vi "2D Array to Excel 2012.vi"   [LabVIEW 2012]
uses:
  <vilib>/Utility/NIReport.llb/NI_report.lvclass
  <vilib>/Utility/NIReport.llb/Excel/NI_Excel.lvclass
  <vilib>/Utility/NIReport.llb/Append Numeric Table to Report (wrap).vi
types:
  T1 = enum16{"Standard Report", "HTML", "Word", "Excel"}
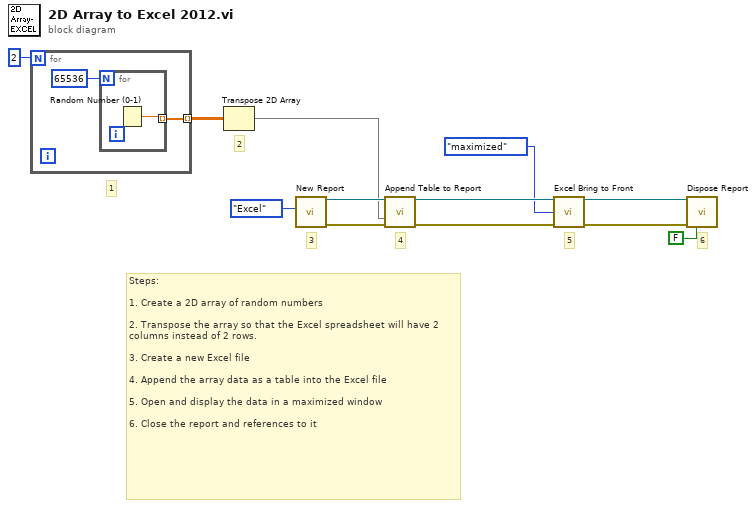
[diagram p0: block diagram]
diagram:
  # "6"
  # "5"
  # "4"
  # "3"
  # "2"
  # "1"
  # "Steps:\n\n1. Create a 2D array of random numbers\n\n2. Transpose the array so that the Excel spreadsheet will have 2 \ncolumns instead of 2 rows.\n\n3. Create a new Excel file\n\n4. Append the array data as a table into the Excel file\n\n5. Open and display the data in a maximized window\n\n6. Close the report and references to it"
  n1 = for {
    N: 2 ("Numeric") -> [_]
    tunnel: [w14] -> w2 mode=indexing
    n2 = for {
      N: 65536 -> [_]
      tunnel: [w15] -> w14 mode=indexing
      n3 = Random Number (0-1)() -> (number: 0 to 1=w15:dbl)
    }
  }
  n4 = Transpose 2D Array(2D array=w2) -> (transposed array=w1:dbl[][])
  n5 = call <vilib>:"New Report.vi"("report type"=T1."Excel") -> ("report out"=w10:refnum<class "NI_report.lvclass">, "error out"=w9:errorcluster)  [unwired: 5 in, 8 out]
  n6 = call-poly <vilib>:"Append Table to Report.vi"("report in"=w10, "numerical data"=w1, "error in (no error)"=w9) -> ("report out"=w7:refnum<class "NI_report.lvclass">, "error out"=w6:errorcluster)  [unwired: 7 in, 4 out]
  n7 = call <vilib>:"Excel Bring to Front.vi"("report in"=w7, "window state (maximized)"=enum16{"maximized", "minimized", "normal"}."maximized", "error in (no error)"=w6) -> ("report out"=w4:refnum<class "NI_report.lvclass">, "error out"=w5:errorcluster)  [unwired: 11 out]
  n8 = call-dynamic "Dispose Report.vi"("report in"=w4, "error in (no error)"=w5, "close report? (T)"=FALSE) -> ()  [unwired: 2 in, 11 out]
